vi "Publish.vi"(7 "headers":string, 8 "error in":errorcluster, 9 "payload":string, 10 "subject":string, 11 "NATS Client.lvlib:NATS Client.lvclass":refnum<class "NATS Client.lvclass">) -> (0 "error out":errorcluster)   [LabVIEW 2024, in "NATS Client.lvlib" / "NATS Client.lvclass"]
doc: "Publishes subject through NATS Client."
uses:
  NATS Client.lvclass
  <vilib>/NATS/NATS Core/VIs/subVIs/Set Timeout.vi
  <vilib>/dlg_ctls.llb/Space Constant.vi
  <vilib>/NATS/NATS Core/NATS Core.lvlib
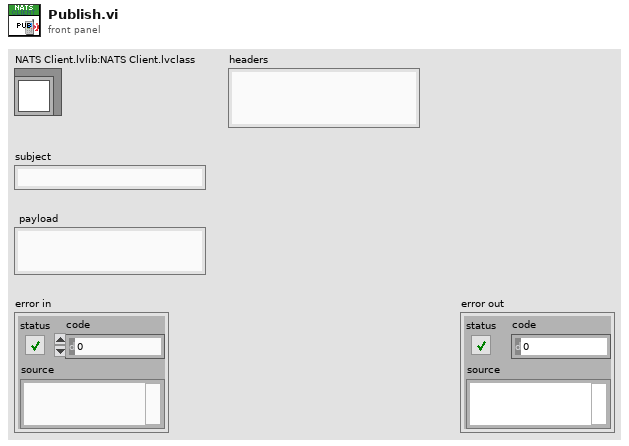
[diagram p1: front panel]
types:
  T1 = typedef "NATS Core.lvlib/nats connection.ctl" = cluster{"connection ID":refnum<k5>, "server INFO":string, "timeout ms":i32, "verbose?":bool, "server headers?":bool, "client headers?":bool}
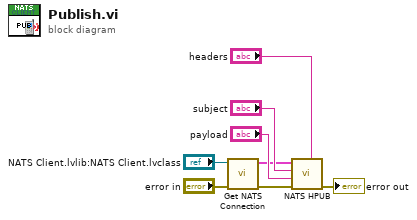
[diagram p0: block diagram]
diagram:
  n1 = call "Get NATS Connection.vi"("error in"="error in", "NATS Client.lvlib:NATS Client.lvclass"="NATS Client.lvlib:NATS Client.lvclass") -> ("error out"=w3:errorcluster, "NATS Connection"=w2:T1)  [unwired: 8 in]
  n2 = call <vilib>:"NATS HPUB.vi"("headers"="headers", "error in"=w3, "payload"="payload", "subject"="subject", "nats connection in"=w2) -> ("error out"=→"error out":errorcluster)  [unwired: 5 in, 1 out]
